vi "Simple Lift Manager.vi"(10 "Numeric":dbl) -> ()   [LabVIEW 2014]
uses:
  Robot Global Data.vi
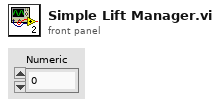
[diagram p1: front panel]
types:
  T1 = typedef "WPI_EncoderDevRef.ctl" = cluster{"DevStatus":errorcluster, "EncoderIndex":T2, "CounterIndex":T3, "DistancePerCount":dbl, "Decoding Type":T4}
  T2 = typedef "FPGA_EncoderIdx.ctl" = enum8{"Enc 0", "Enc 1", "Enc 2", "Enc 3", "Enc 4", "Enc 5", "Enc 6", "Enc 7", "Invalid"}
  T3 = typedef "FPGA_CounterCtrSystemIndex.ctl" = enum8{"Ctr 0", "Ctr 1", "Ctr 2", "Ctr 3", "Ctr 4", "Ctr 5", "Ctr 6", "Ctr 7", "Invalid"}
  T4 = typedef "WPI_EncoderType.ctl" = enum16{"1x", "2x", "4x"}
  T5 = typedef "WPI_DigitalInputDevRef.ctl" = cluster{"DevStatus":errorcluster, "DIO Channel":T6, "Controller":T7}
  T6 = typedef "FPGA_DIOChannel.ctl" = enum8{"DIO 0", "DIO 1", "DIO 2", "DIO 3", "DIO 4", "DIO 5", "DIO 6", "DIO 7", "DIO 8", "DIO 9", "DIO MXP 0", "DIO MXP 1", "DIO MXP 2", "DIO MXP 3", "DIO MXP 4", "DIO MXP 5", "DIO MXP 6", "DIO MXP 7", "DIO MXP 8", "DIO MXP 9", "DIO MXP 10", "DIO MXP 11", "DIO MXP 12", "DIO MXP 13", "DIO MXP 14", "DIO MXP 15", "Invalid"}
  T7 = typedef "FPGA_TypedefDigitalModule.ctl" = enum16{"Controller 1"}
  T8 = typedef "WPI_MotorControlDeviceRef.ctl" = cluster{"DeviceStatus":errorcluster, "Type":T9, "PWM":cluster{"Controller":T7, "PWM Channel":T10, "DeadBand":T11}, "CAN":cluster{"Device Number":u8, "Control Mode":T12, "Semaphore":T13, "Max Vout":dbl, "TalonSRX Control Mode":T14}, "Invert":bool, "TransformRef":T15, "InvTransformRef":T15}
  T9 = typedef "WPI_MotorControlType.ctl" = enum16{"PWM", "CAN", "CANTalonSRX"}
  T10 = typedef "FPGA_DIOPWMChannel.ctl" = enum8{"PWM 0", "PWM 1", "PWM 2", "PWM 3", "PWM 4", "PWM 5", "PWM 6", "PWM 7", "PWM 8", "PWM 9", "PWM MXP 0", "PWM MXP 1", "PWM MXP 2", "PWM MXP 3", "PWM MXP 4", "PWM MXP 5", "PWM MXP 6", "PWM MXP 7", "PWM MXP 8", "PWM MXP 9", "Invalid"}
  T11 = typedef "WPI_PWMDeadband.ctl" = cluster{"Name":string, "maxPositivePwm":i32, "minPositivePwm":i32, "centerPwm":i32, "maxNegativePwm":i32, "minNegativePwm":i32, "angularRange":u16}
  T12 = typedef "WPI_CANJaguar_ControlMode.ctl" = enum8{"Percent VBus", "Current", "Speed", "Position", "Voltage"}
  T13 = typedef "Semaphore RefNum" = refnum<k1>
  T14 = typedef "WPI_CANTalonSRX_APIControlMode.ctl" = enum8{"Percent VBus", "Speed", "Position", "Slave", "Unchanged / Invalid"}
  T15 = typedef "WPI_PWMTransform_ConPane.ctl" = refnum<vi>
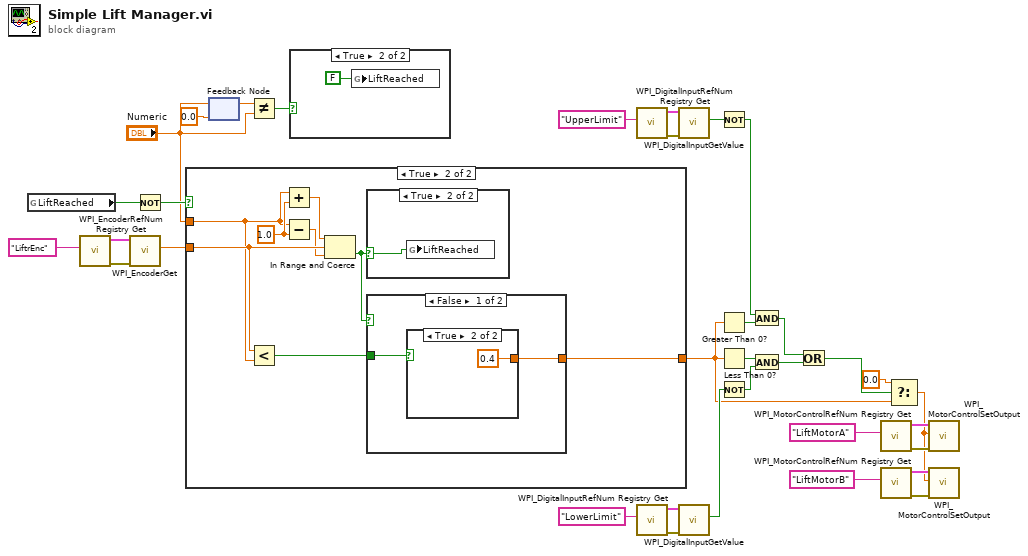
[diagram p0: block diagram]
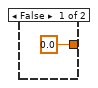
[diagram p2: hidden frame]
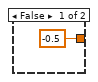
[diagram p4: hidden frame]
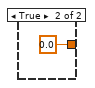
[diagram p5: hidden frame]
diagram:
  n1 = global read "Robot Global Data.vi" "LiftReached"() -> (w7:bool)
  n2 = call <vilib>:"WPI_EncoderRefNum Registry Get.vi"("refnum name"="LiftrEnc") -> ("error out"=w33:errorcluster, "EncoderDevRef"=w32:T1)  [unwired: 9 in]
  n3 = call <vilib>:"WPI_EncoderGet.vi"("error in (no error)"=w33, "EncoderDevRef"=w32) -> ("Distance"=w11:dbl)  [unwired: 4 in, 5 out]
  n4 = Not(x=w7) -> (.not. x?=w6:bool)
  n5 = case shown="True" w6 {
    tunnel: [0.0 w43] -> w12
    tunnel: w11 -> [_ w41]
    tunnel: "Numeric" -> [_ w36]
    frame False {
    }
    frame True {
      w38 = 1.0
      n6 = Less?(x=w41, y=w36) -> (x < y?=w42:bool)
      n7 = Add(x=w36, y=w38) -> (x+y=w40:dbl)
      n8 = Subtract(x=w36, y=w38) -> (x-y=w39:dbl)
      n9 = In Range and Coerce(upper limit=w40, x=w41, lower limit=w39) -> (In Range?=w37:bool)  [unwired: 1 out]
      n10 = case shown="True" w37 {
        selector: w37 -> [_ w44]
        frame False {
        }
        frame True {
          n11 = global write "Robot Global Data.vi" "LiftReached"(w44) -> ()
        }
      }
      n12 = case shown="False" w37 {
        tunnel: [w45 0.0] -> w43
        tunnel: w42 -> [w46 _]
        frame False {
          n13 = case shown="True" w46 {
            tunnel: [-0.5 0.4] -> w45
            frame False {
            }
            frame True {
            }
          }
        }
        frame True {
        }
      }
    }
  }
  n14 = feedback #1(0.0) -> (w9:dbl)
  n15 = feedback-in #1("Numeric") -> ()
  n16 = Not Equal?(x=w9, y="Numeric") -> (x != y?=w8:bool)
  n17 = case shown="True" w8 {
    frame False {
    }
    frame True {
      n18 = global write "Robot Global Data.vi" "LiftReached"(FALSE) -> ()
    }
  }
  n19 = call <vilib>:"WPI_DigitalInputRefNum Registry Get.vi"("refnum name"="UpperLimit") -> ("error out"=w20:errorcluster, "DigitalInputDevRef"=w19:T5)  [unwired: 9 in]
  n20 = call <vilib>:"WPI_DigitalInputRefNum Registry Get.vi"("refnum name"="LowerLimit") -> ("error out"=w18:errorcluster, "DigitalInputDevRef"=w17:T5)  [unwired: 9 in]
  n21 = call <vilib>:"WPI_DigitalInputGetValue.vi"("error in (no error)"=w20, "DigitalInputDevRef"=w19) -> ("Value"=w14:bool)  [unwired: 7 in, 2 out]
  n22 = call <vilib>:"WPI_DigitalInputGetValue.vi"("error in (no error)"=w18, "DigitalInputDevRef"=w17) -> ("Value"=w13:bool)  [unwired: 7 in, 2 out]
  n23 = Not(x=w14) -> (.not. x?=w23:bool)
  n24 = Greater Than 0?(x=w12) -> (x > 0?=w26:bool)
  n25 = Less Than 0?(x=w12) -> (x < 0?=w25:bool)
  n26 = Not(x=w13) -> (.not. x?=w24:bool)
  n27 = And(x=w23, y=w26) -> (x .and. y?=w22:bool)
  n28 = And(x=w25, y=w24) -> (x .and. y?=w21:bool)
  n29 = Or(x=w22, y=w21) -> (x .or. y?=w28:bool)
  n30 = call <vilib>:"WPI_MotorControlRefNum Registry Get.vi"("refnum name"="LiftMotorA") -> ("error out"=w30:errorcluster, "MotorControlDevRef"=w29:T8)  [unwired: 9 in]
  n31 = call <vilib>:"WPI_MotorControlRefNum Registry Get.vi"("refnum name"="LiftMotorB") -> ("error out"=w3:errorcluster, "MotorControlDevRef"=w2:T8)  [unwired: 9 in]
  n32 = Select(t=0.0, s=w28, f=w12) -> (s? t:f=w1:dbl)
  n33 = call <vilib>:"WPI_MotorControlSetOutput.vi"("error in (no error)"=w30, "Output"=w1, "MotorControlDevRef"=w29) -> ()  [unwired: 6 in, 3 out]
  n34 = call <vilib>:"WPI_MotorControlSetOutput.vi"("error in (no error)"=w3, "Output"=w1, "MotorControlDevRef"=w2) -> ()  [unwired: 6 in, 3 out]
